vi "Intan_UpdateMarkers.vi"(0 "Free Select Chans":bool=TRUE, 1 "Picture In":picture, 2 "Display Chans":i32[](listbox)=[1, 4, 13, 14, 15, 16, 17, 22], 3 "plot bounds":T1, 4 "YtxtLabelsAll":string[](array[string])) -> (5 "Picture Out":picture, 6 "update labels":bool)   [LabVIEW 2015]
uses:
  <vilib>/Utility/miscctls.llb/LVRectTypeDef.ctl
panel:
  out "Picture":picture
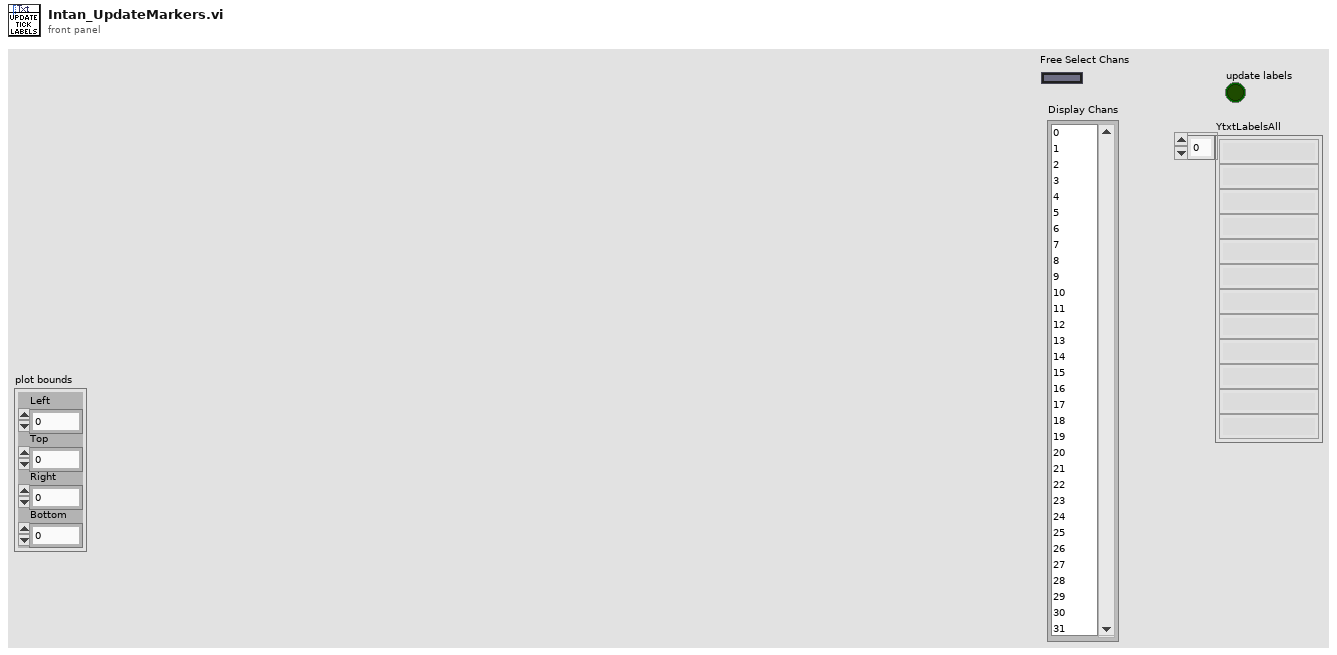
[diagram p1: front panel]
types:
  T1 = typedef "LVRectTypeDef.ctl" = cluster{"Left":i16, "Top":i16, "Right":i16, "Bottom":i16}
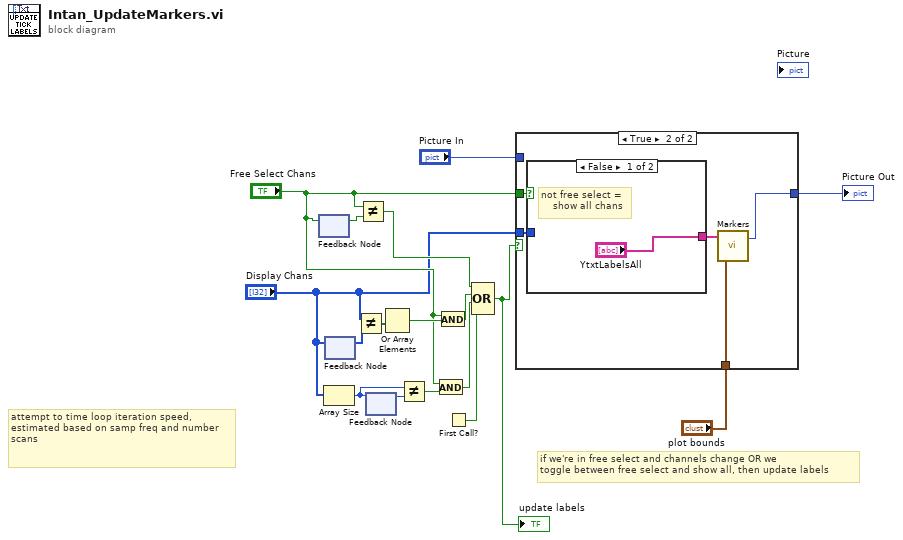
[diagram p0: block diagram]
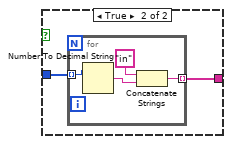
[diagram p3: hidden frame]
diagram:
  # "if we're in free select and channels change OR we\ntoggle between free select and show all, then update labels"
  # "attempt to time loop iteration speed,\nestimated based on samp freq and number scans"
  n1 = feedback #1() -> (w12:bool)  [unwired: 1 in]
  n2 = feedback-in #1("Free Select Chans") -> ()
  n3 = Array Size(array="Display Chans") -> (size(s)=w11:i32)
  n4 = feedback #2() -> (w16:i32[])  [unwired: 1 in]
  n5 = feedback-in #2("Display Chans") -> ()
  n6 = Not Equal?(x="Display Chans", y=w16) -> (x != y?=w15:bool[])
  n7 = Not Equal?(x="Free Select Chans", y=w12) -> (x != y?=w13:bool)
  n8 = feedback #3() -> (w10:i32)  [unwired: 1 in]
  n9 = feedback-in #3(w11) -> ()
  n10 = Or Array Elements(Boolean array=w15) -> (logical OR=w17:bool)
  n11 = Not Equal?(x=w11, y=w10) -> (x != y?=w9:bool)
  n12 = And(x="Free Select Chans", y=w9) -> (x .and. y?=w8:bool)
  n13 = And(x="Free Select Chans", y=w17) -> (x .and. y?=w14:bool)
  n14 = First Call?() -> (First Call?: T/F=w7:bool)
  n15 = Compound Arithmetic op=OR(w13, w14, w8, w7) -> (w4:bool)
  "update labels" <- w4
  n16 = case shown="True" w4 {
    tunnel: "Free Select Chans" -> [_ w22]
    tunnel: "Display Chans" -> [_ w21]
    tunnel: "plot bounds" -> [_ w20]
    tunnel: [w18 w19] -> w2
    tunnel: "Picture In" -> [w18 _]
    frame False {
    }
    frame True {
      n17 = case shown="False" w22 {
        tunnel: w21 -> [_ w26]
        tunnel: ["YtxtLabelsAll" w25] -> w23
        frame False {
          # "not free select = \n    show all chans"
        }
        frame True {
          n18 = for {
            tunnel: w26 -> [w30] mode=indexing
            tunnel: [w27] -> w25 mode=indexing
            n19 = Number To Decimal String(number=w30) -> (decimal integer string=w29:string)  [unwired: 1 in]
            n20 = Concatenate Strings("in" ("string"), w29) -> (w27:string)
          }
        }
      }
      n21 = call "Markers.vi"("plot bounds"=w20, "Array"=w23) -> ("Picture"=w19:picture)  [unwired: 1 out]
    }
  }
  "Picture Out" <- w2
